vi "L11.vi"() -> ()   [LabVIEW 2012]
panel:
  out "Intensity Graph 3":i64[][](graph)
  out "Intensity Graph 2":i64[][](graph)
  out "product":i64
  out "Intensity Graph 4":i64[][](graph)
  out "Intensity Graph 1":i64[][](graph)
  out "array":dbl[][](array[numeric])
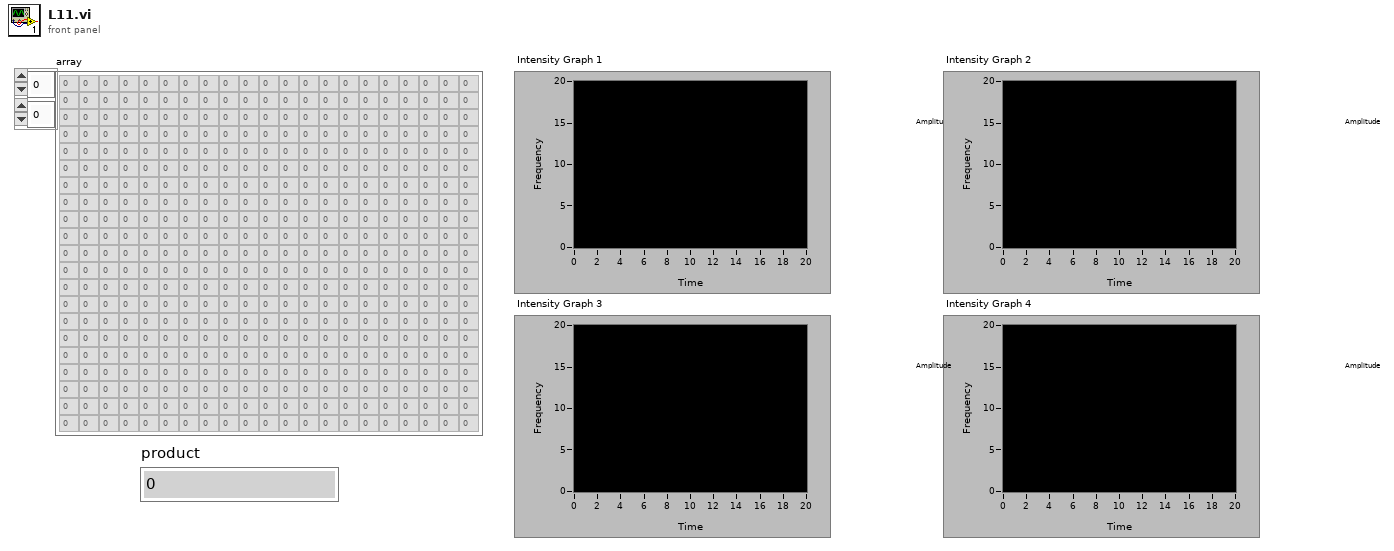
[diagram p1: front panel]
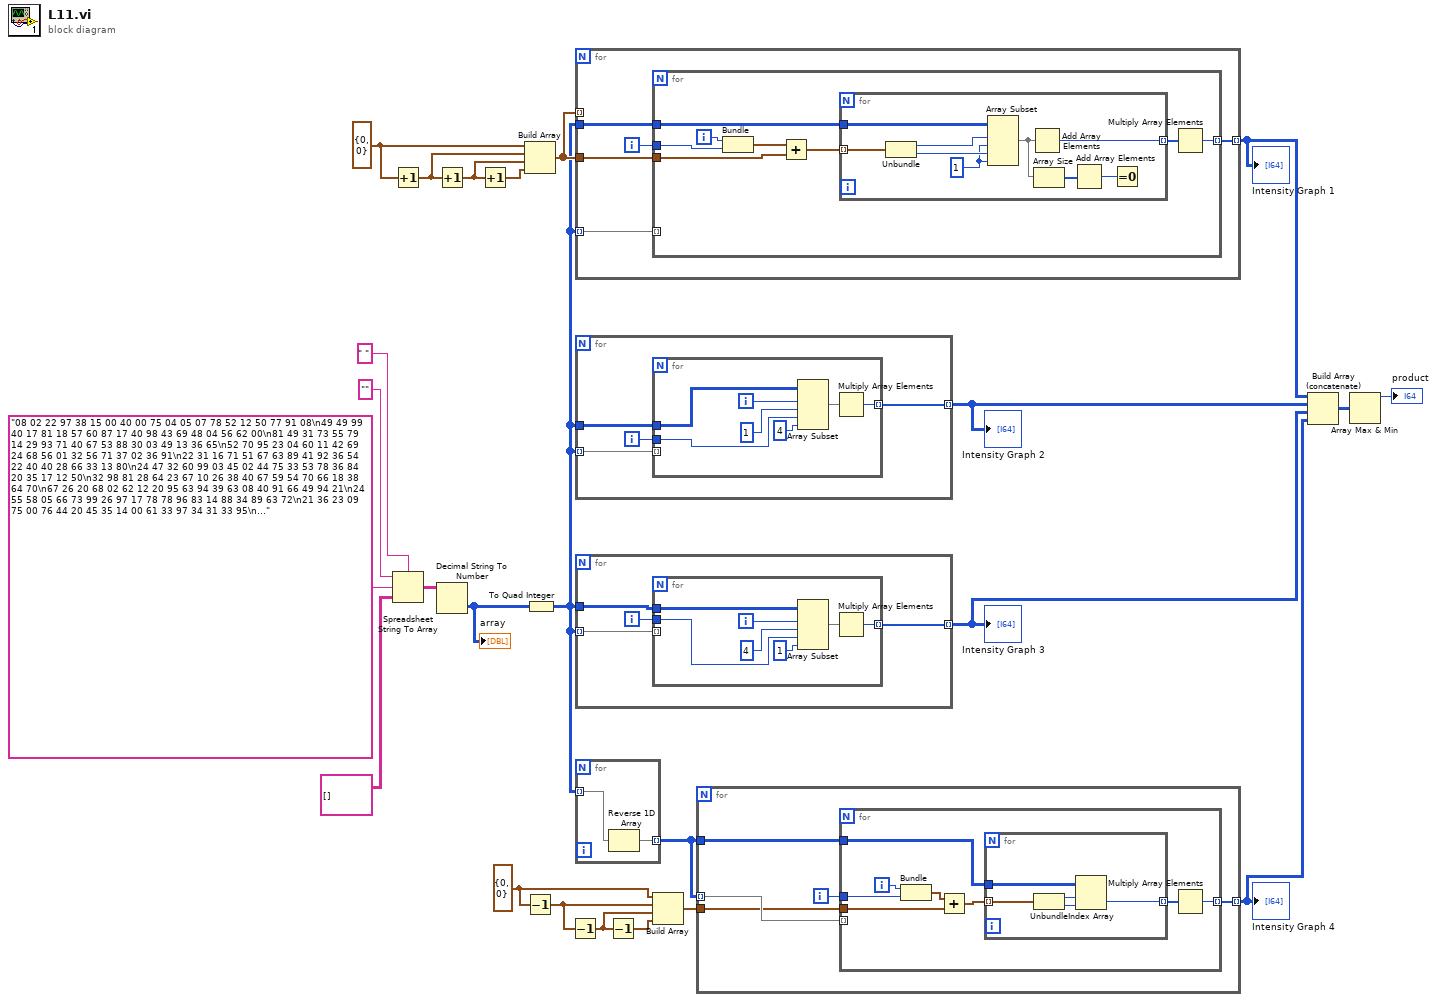
[diagram p0: block diagram]
diagram:
  w11 = cluster{i32, i32} {0, 0} ("output cluster")
  w19 = cluster{i32, i32} {0, 0} ("output cluster")
  n1 = Increment(x=w19) -> (x+1=w18:cluster{i32, i32})
  n2 = Spreadsheet String To Array(delimiter (Tab)=" ", format string="" ("spreadsheet string"), spreadsheet string="08 02 22 97 38 15 00 40 00 75 04 05 07 78 52 12 50 77 91 08\n49 49 99 40 17 81 18 57 60 87 17 40 98 43 69 48 04 56 62 00\n81 49 31 73 55 79 14 29 93 71 40 67 53 88 30 03 49 13 36 65\n52 70 95 23 04 60 11 42 69 24 68 56 01 32 56 71 37 02 36 91\n22 31 16 71 51 67 63 89 41 92 36 54 22 40 40 28 66 33 13 80\n24 47 32 60 99 03 45 02 44 75 33 53 78 36 84 20 35 17 12 50\n32 98 81 28 64 23 67 10 26 38 40 67 59 54 70 66 18 38 64 70\n67 26 20 68 02 62 12 20 95 63 94 39 63 08 40 91 66 49 94 21\n24 55 58 05 66 73 99 26 97 17 78 78 96 83 14 88 34 89 63 72\n21 36 23 09 75 00 76 44 20 45 35 14 00 61 33 97 34 31 33 95\n78 17 53 28 22 75 31 67 15 94 03 80 04 62 16 14 09 53 56 92\n16 39 05 42 96 35 31 47 55 58 88 24 00 17 54 24 36 29 85 57\n86 56 00 48 35 71 89 07 05 44 44 37 44 60 21 58 51 54 17 58\n19 80 81 68 05 94 47 69 28 73 92 13 86 52 17 77 04 89 55 40\n04 52 08 83 97 35 99 16 07 97 57 32 16 26 26 79 33 27 98 66\n88 36 68 87 57 62 20 72 03 46 33 67 46 55 12 32 63 93 53 69\n04 42 16 73 38 25 39 11 24 94 72 18 08 46 29 32 40 62 76 36\n20 69 36 41 72 30 23 88 34 62 99 69 82 67 59 85 74 04 36 16\n20 73 35 29 78 31 90 01 74 31 49 71 48 86 81 16 23 57 05 54\n01 70 54 71 83 51 54 69 16 92 33 48 61 43 52 01 89 19 67 48", array type (2D Dbl)=string[][] []) -> (array=w20:string[][])
  n3 = Increment(x=w18) -> (x+1=w17:cluster{i32, i32})
  n4 = Decimal String To Number(string=w20) -> (number=w3:i32[][])  [unwired: 2 in, 1 out]
  "array" <- w3
  n5 = Increment(x=w17) -> (x+1=w16:cluster{i32, i32})
  n6 = Build Array(w19, w18, w17, w16) -> (w2:cluster{i32, i32}[])
  n7 = Decrement(x=w11) -> (x-1=w12:cluster{i32, i32})
  n8 = To Quad Integer(1:w3) -> (0:w1:i64[][])
  n9 = Decrement(x=w12) -> (x-1=w13:cluster{i32, i32})
  n10 = for {
    tunnel: w1 -> [w29]
    tunnel: w1 -> [w28] mode=indexing
    tunnel: w2 -> [w26]
    tunnel: [w25] -> w10 mode=indexing
    tunnel: w2 -> [_] mode=indexing
    i -> [w27]
    n11 = for {
      tunnel: w29 -> [w37]
      tunnel: w28 -> [_] mode=indexing
      tunnel: w27 -> [w35]
      tunnel: w26 -> [w33]
      tunnel: [w30] -> w25 mode=indexing
      i -> [w36]
      n12 = Bundle(w36, w35) -> (w34:cluster{i32, i32})  [unwired: 1 in]
      n13 = Add(x=w34, y=w33) -> (x+y=w32:cluster{i32, i32}[])
      n14 = for {
        tunnel: w37 -> [w45]
        tunnel: w32 -> [w46] mode=indexing
        tunnel: [w41] -> w31 mode=indexing
        w42 = 1 ("length")
        n15 = Unbundle(w46) -> (w44:i32, w43:i32)
        n16 = Array Subset(array=w45, index (row)=w44, length (row)=w42, index (col)=w43, length (col)=w42) -> (w40:i64[][])
        n17 = Add Array Elements(numeric array=w40) -> (sum=w41:i64)
        n18 = Array Size(array=w40) -> (size(s)=w39:i32[])
        n19 = Add Array Elements(numeric array=w39) -> (sum=w38:i32)
        n20 = Equal To 0?(x=w38) -> ()  [unwired: 1 out]
      }
      n21 = Multiply Array Elements(1:w31) -> (0:w30:i64)
    }
  }
  "Intensity Graph 1" <- w10
  n22 = for {
    tunnel: w1 -> [w50]
    tunnel: w1 -> [w49] mode=indexing
    tunnel: [w47] -> w5 mode=indexing
    i -> [w48]
    n23 = for {
      tunnel: w50 -> [w57]
      tunnel: w49 -> [_] mode=indexing
      tunnel: w48 -> [w55]
      tunnel: [w51] -> w47 mode=indexing
      i -> [w56]
      n24 = Array Subset(array=w57, index (row)=w56, length (row)=1 ("length"), index (col)=w55, length (col)=4 ("length")) -> (w52:i64[][])
      n25 = Multiply Array Elements(1:w52) -> (0:w51:i64)
    }
  }
  "Intensity Graph 2" <- w5
  n26 = for {
    tunnel: w1 -> [w61]
    tunnel: w1 -> [w60] mode=indexing
    tunnel: [w58] -> w4 mode=indexing
    i -> [w59]
    n27 = for {
      tunnel: w61 -> [w68]
      tunnel: w60 -> [_] mode=indexing
      tunnel: w59 -> [w66]
      tunnel: [w62] -> w58 mode=indexing
      i -> [w67]
      n28 = Array Subset(array=w68, index (row)=w67, length (row)=4 ("length"), index (col)=w66, length (col)=1 ("length")) -> (w63:i64[][])
      n29 = Multiply Array Elements(1:w63) -> (0:w62:i64)
    }
  }
  "Intensity Graph 3" <- w4
  n30 = for {
    tunnel: w1 -> [w70] mode=indexing
    tunnel: [w69] -> w6 mode=indexing
    n31 = Reverse 1D Array(array=w70) -> (reversed array=w69:i64[])
  }
  n32 = Decrement(x=w13) -> (x-1=w14:cluster{i32, i32})
  n33 = Build Array(w11, w12, w13, w14) -> (w15:cluster{i32, i32}[])
  n34 = for {
    tunnel: w6 -> [w75]
    tunnel: w6 -> [w74] mode=indexing
    tunnel: w15 -> [w72]
    tunnel: [w71] -> w7 mode=indexing
    i -> [w73]
    n35 = for {
      tunnel: w75 -> [w83]
      tunnel: w74 -> [_] mode=indexing
      tunnel: w73 -> [w81]
      tunnel: w72 -> [w79]
      tunnel: [w76] -> w71 mode=indexing
      i -> [w82]
      n36 = Bundle(w82, w81) -> (w80:cluster{i32, i32})  [unwired: 1 in]
      n37 = Add(x=w80, y=w79) -> (x+y=w78:cluster{i32, i32}[])
      n38 = for {
        tunnel: w83 -> [w88]
        tunnel: w78 -> [w87] mode=indexing
        tunnel: [w84] -> w77 mode=indexing
        n39 = Unbundle(w87) -> (w86:i32, w85:i32)
        n40 = Index Array "Index Array"(array=w88, index (row)=w86, index (col)=w85) -> (element=w84:i64)
      }
      n41 = Multiply Array Elements(1:w77) -> (0:w76:i64)
    }
  }
  "Intensity Graph 4" <- w7
  n42 = Build Array (concatenate)(w10, w5, w4, w7) -> (w9:i64[][])
  n43 = Array Max & Min(array=w9) -> (max value=→"product":i64)  [unwired: 3 out]
